vi "hydraharp_write_header.vi"(8 "error in (no error)":errorcluster, 11 "hydraharp in":refnum<class "hydraharp.lvclass">) -> (0 "error out":errorcluster, 3 "hydraharp out":refnum<class "hydraharp.lvclass">)   [LabVIEW 2015, in "hydraharp.lvclass"]
uses:
  hydraharp.lvclass
  hydraharp.lvclass/hydraharp.ctl
  hdf5_photon_record_logger/stream_metadata.ctl
  hydraharp_panel/hpanel_hydraharp_settings.ctl
  hydraharp_panel/hpanel_sync_settings.ctl
  hydraharp_panel/hpanel_sync_div.ctl
  hydraharp_panel/hpanel_channel_settings.ctl
  Data Logger Class/data_logger.lvclass
  hhlib.dll
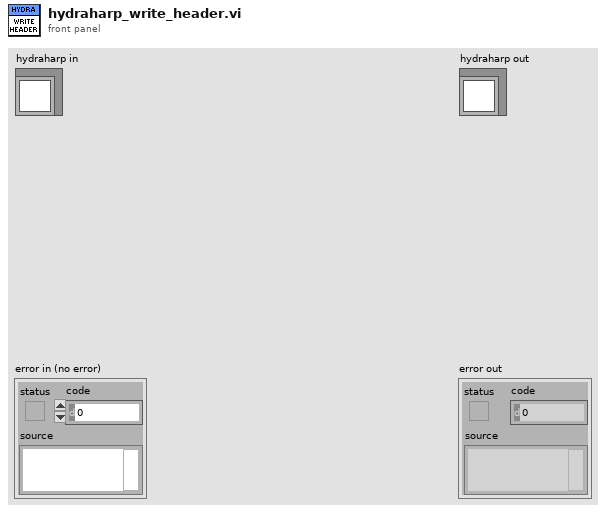
[diagram p1: front panel]
types:
  T1 = typedef "stream_metadata.ctl" = cluster{"Hydraharp Settings":T2, "resolution":dbl, "stream_notes":string}
  T2 = typedef "hpanel_hydraharp_settings.ctl" = cluster{"Sync Settings":T3, "CH 1":T5, "CH 2":T5, "CH 3":T5, "CH 4":T5, "binning":i32, "CH 5":T5, "CH 6":T5, "CH 7":T5, "CH 8":T5}
  T3 = typedef "hpanel_sync_settings.ctl" = cluster{"snc_count":i32, "snc_level":i32, "snc_ZeroX":i32, "snc_offs":i32, "sync_div":T4}
  T4 = typedef "hpanel_sync_div.ctl" = enum16{"1", "2", "4", "8"}
  T5 = typedef "hpanel_channel_settings.ctl" = cluster{"ch_counts":i32, "ch_level":i32, "ch_ZeroX":i32, "ch_offs":i32}
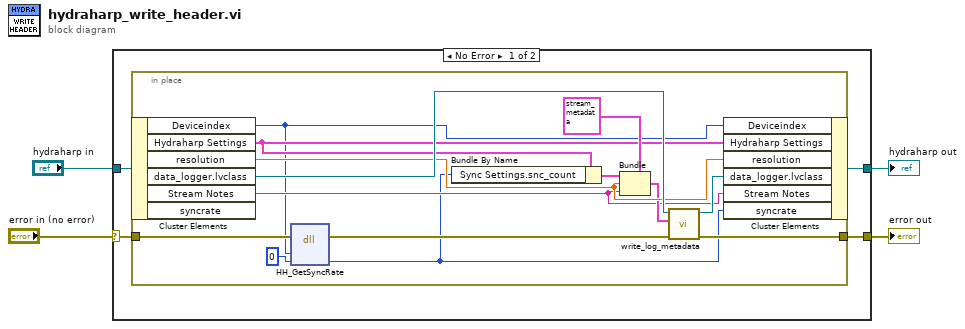
[diagram p0: block diagram]
diagram:
  n1 = case shown="No Error" "error in (no error)" {
    selector: "error in (no error)" -> [w8 w24]
    tunnel: [w5 w24] -> w3
    tunnel: [w6 w23] -> w1
    tunnel: "hydraharp in" -> [w7 w23]
    frame No Error {
      n2 = in-place {
        in-place-border: w8 -> [w13]
        in-place-border: [w18] -> w5
        n3 = in-place-cluster #1(w7) -> ("Deviceindex"=w9:i32, "Hydraharp Settings"=w14:T2, "resolution"=w20:dbl, "data_logger.lvclass"=w22:refnum<class "data_logger.lvclass">, "Stream Notes"=w17:string)  [unwired: 1 out]
        n4 = dll-call lib="hhlib.dll" fn="HH_GetSyncRate"(error in=w13, "devidx"=w9, "syncrate"=0) -> (error out=w12:errorcluster, "syncrate"=w10:i32)  [unwired: 4 in, 1 out]
        n5 = Bundle By Name(cluster=w14, "Sync Settings.snc_count"=w10) -> (w15:T2)
        n6 = Bundle(cluster=T1 {"Hydraharp Settings"={"Sync Settings"={"snc_count"=0, "snc_level"=0, "snc_ZeroX"=0, "snc_offs"=0, "sync_div"=enum."1"}, "CH 1"={"ch_counts"=0, "ch_level"=0, "ch_ZeroX"=0, "ch_offs"=0}, "CH 2"={"ch_counts"=0, "ch_level"=0, "ch_ZeroX"=0, "ch_offs"=0}, "CH 3"={"ch_counts"=0, "ch_level"=0, "ch_ZeroX"=0, "ch_offs"=0}, "CH 4"={"ch_counts"=0, "ch_level"=0, "ch_ZeroX"=0, "ch_offs"=0}, "binning"=0, "CH 5"={"ch_counts"=0, "ch_level"=0, "ch_ZeroX"=0, "ch_offs"=0}, "CH 6"={"ch_counts"=0, "ch_level"=0, "ch_ZeroX"=0, "ch_offs"=0}, "CH 7"={"ch_counts"=0, "ch_level"=0, "ch_ZeroX"=0, "ch_offs"=0}, "CH 8"={"ch_counts"=0, "ch_level"=0, "ch_ZeroX"=0, "ch_offs"=0}}, "resolution"=0.0, "stream_notes"="stream_notes"} ("output cluster"), "Hydraharp Settings"=w15, "resolution"=w20, "stream_notes"=w17) -> (w19:T1)
        n7 = call-dynamic "write_log_metadata.vi"("error in (no error)"=w12, "data"=w19, "data_logger in"=w22) -> ("error out"=w18:errorcluster, "data_logger out"=w21:refnum<class "data_logger.lvclass">)  [unwired: 7 in]
        n8 = in-place-cluster #1("Deviceindex"=w9, "Hydraharp Settings"=w14, "resolution"=w20, "data_logger.lvclass"=w21, "Stream Notes"=w17, "syncrate"=w10) -> (w6:refnum<class "hydraharp.lvclass">)
      }
    }
    frame Error {
    }
  }
  "error out" <- w3
  "hydraharp out" <- w1
